vi "Material-Dialog-UnloadSheet.vi"(8 "error in (no error)":errorcluster) -> (0 "error out":errorcluster)   [LabVIEW 2013, in "Material-RunTest.lvclass"]
uses:
  Material-RunTest.lvclass
panel:
  in  "Finished":bool
  out "String":string="Remove the sheet of Material off the chuck now."
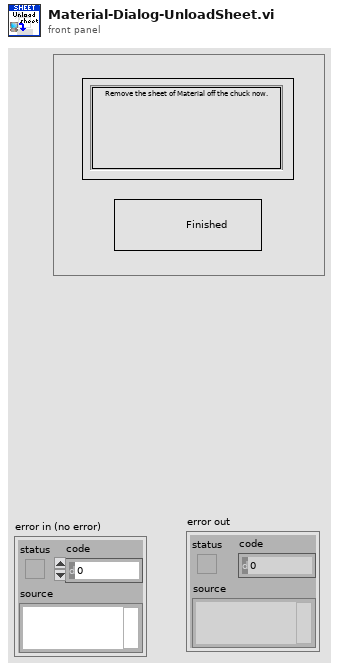
[diagram p1: front panel]
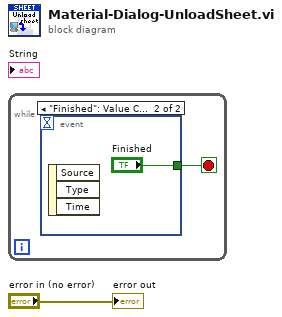
[diagram p0: block diagram]
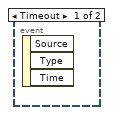
[diagram p2: hidden frame]
diagram:
  n1 = while {
    stop <- w2 stop-if-true
    n2 = event shown="[1] \"Finished\": Value Change" {
      selector: _ -> [_ _]
      dyn-events: _ -> [_ _]
      timeout: _ -> [_ _]
      tunnel: [_ "Finished"] -> w2
      event Timeout {
        n3 = event-data() -> ()  [unwired: 1 in, 3 out]
      }
      event "Finished": Value Change {
        n4 = event-data() -> ()  [unwired: 1 in, 3 out]
      }
    }
  }
  "error out" <- "error in (no error)"
